vi "1_1.vi"() -> ()   [LabVIEW 2020]
panel:
  out "String":string
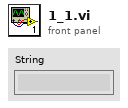
[diagram p1: front panel]
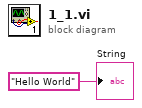
[diagram p0: block diagram]
diagram:
  "String" <- "Hello World" ("String")
